vi "rvc Create Link.vi"(11 "rotation angle (theta)":dbl) -> (3 "output cluster":T1)   [LabVIEW 2013]
uses:
  <vilib>/robotics/Kinematics/Link/Joint Type.ctl
  <vilib>/robotics/Kinematics/Link/NI_Robotics_Link.lvclass
  <vilib>/robotics/Kinematics/DH Kinematic Parameters.ctl
panel:
  in  "offset distance":dbl
  in  "length (d)":dbl
  in  "twist angle (alpha)":dbl
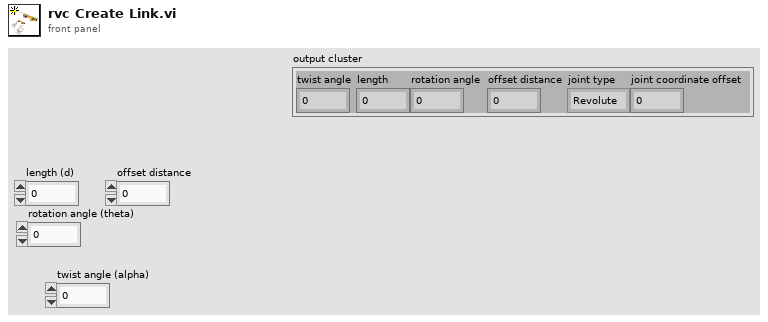
[diagram p1: front panel]
types:
  T1 = typedef "DH Kinematic Parameters.ctl" = cluster{"twist angle":dbl, "length":dbl, "rotation angle":dbl, "offset distance":dbl, "joint type":T2, "joint coordinate offset":dbl}
  T2 = typedef "NI_Robotics_Link.lvclass/Joint Type.ctl" = enum16{"Revolute", "Prismatic"}
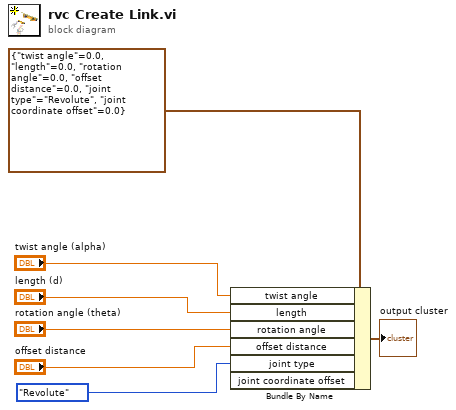
[diagram p0: block diagram]
diagram:
  n1 = Bundle By Name(cluster=T1 {"twist angle"=0.0, "length"=0.0, "rotation angle"=0.0, "offset distance"=0.0, "joint type"=enum."Revolute", "joint coordinate offset"=0.0} ("Link Parameters"), "twist angle"="twist angle (alpha)", "length"="length (d)", "rotation angle"="rotation angle (theta)", "offset distance"="offset distance", "joint type"=Joint_Type."Revolute") -> (→"output cluster":T1)  [unwired: 1 in]
